vi "Planing.vi"(8 "error in (no error)":errorcluster, 10 "Reset":bool) -> (0 "error out":errorcluster)   [LabVIEW 2019]
doc: "Returns the horizontal xy-position of the haptic pen in nm, and the vertical z-position in mm. The horizontal position depends on the frame origin and frame size.\n\n<b>Position:</b> Returns a cluster of the x (nm), y (nm), and z (mm) positions of the pen."
uses:
  dll_path.vi
  Haptic Prog Interface.lvlib
panel:
  in  "Toggle":bool
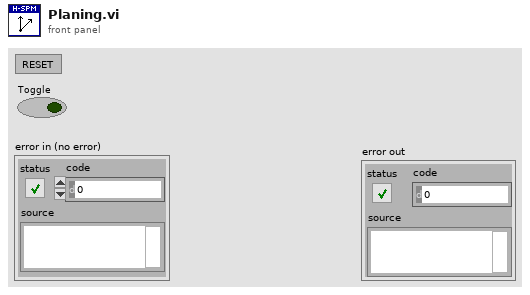
[diagram p1: front panel]
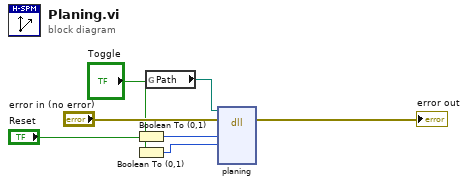
[diagram p0: block diagram]
diagram:
  n1 = Boolean To (0,1)(Boolean="Reset") -> (0, 1=w4:i16)
  n2 = Boolean To (0,1)(Boolean="Toggle") -> (0, 1=w2:i16)
  n3 = global read "dll_path.vi" "Path"() -> (w7:path)
  n4 = dll-call lib="C:/Users/freem/Documents/GitHub/HapticSPM/Haptic-Programming-Interface/x64/Release/Haptic Programming Interface.dll" fn="planing"(path in=w7, error in="error in (no error)", "reset"=w4, "planing"=w2) -> (error out=→"error out":errorcluster)  [unwired: 8 in, 1 out]
